vi "dBm_MeanSD.vi"(0 "dBm array":dbl[](array[numeric])) -> (4 "dBm mean":dbl format="%0.2f", 6 "Std Dev":dbl format="%0.2f")   [LabVIEW 2012]
doc: "The input is an array of power in dBm. The values are linearized -- the mean, standard deviation, and variance are computed - converted back into dBm and returned."
uses:
  <vilib>/Analysis/NI_AALBase.lvlib
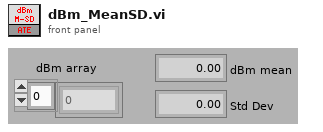
[diagram p1: front panel]
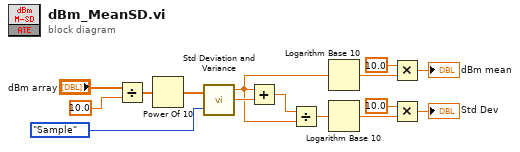
[diagram p0: block diagram]
diagram:
  n1 = Divide(x="dBm array", y=10.0) -> (x/y=w14:dbl[])
  n2 = Power Of 10(x=w14) -> (10^x=w13:dbl[])
  n3 = call <vilib>:"Std Deviation and Variance.vi"("X"=w13, "Weighting (Sample)"=enum16{"Sample", "Population"}."Sample") -> ("mean"=w2:dbl, "standard deviation"=w7:dbl)  [unwired: 1 out]
  n4 = Add(x=w2, y=w7) -> (x+y=w1:dbl)
  n5 = Divide(x=w1, y=w2) -> (x/y=w4:dbl)
  n6 = Logarithm Base 10(1:w2) -> (0:w11:dbl)
  n7 = Logarithm Base 10(1:w4) -> (0:w6:dbl)
  n8 = Multiply(x=10.0, y=w11) -> (x*y=→"dBm mean":dbl)
  n9 = Multiply(x=10.0, y=w6) -> (x*y=→"Std Dev":dbl)
